vi "addBroadcastFreezeSensorValuesFrame.vi"(8 "error in (no error)":errorcluster, 9 "TriggerIRQ":bool, 10 "WaitForTrigger":bool, 11 "Subnet in":refnum<class "Subnet.lvclass">) -> (0 "error out":errorcluster, 3 "Subnet out":refnum<class "Subnet.lvclass">)   [LabVIEW 2016, in "Subnet.lvclass"]
uses:
  Subnet.lvclass
  Subnet.lvclass/Subnet.ctl
  Common_RT_Modbus/IModbus/IModbus.lvclass
  Common_RT_HPILC/HPILC/HPILC.lvclass
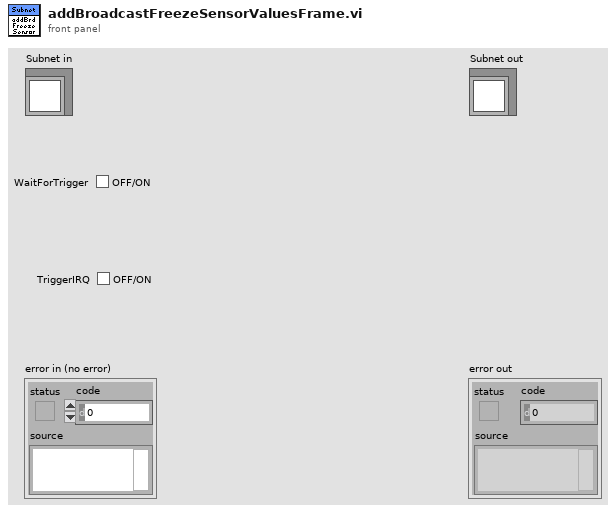
[diagram p1: front panel]
types:
  T1 = typedef "RTModbus.lvlib/TxFrame.ctl" = cluster{"Data":u8[], "WaitForTrigger":bool, "WaitForRx":u16, "TriggerIRQ":bool, "DelayMicroseconds":u16, "DelayMilliseconds":u16, "Timestamp":bool}
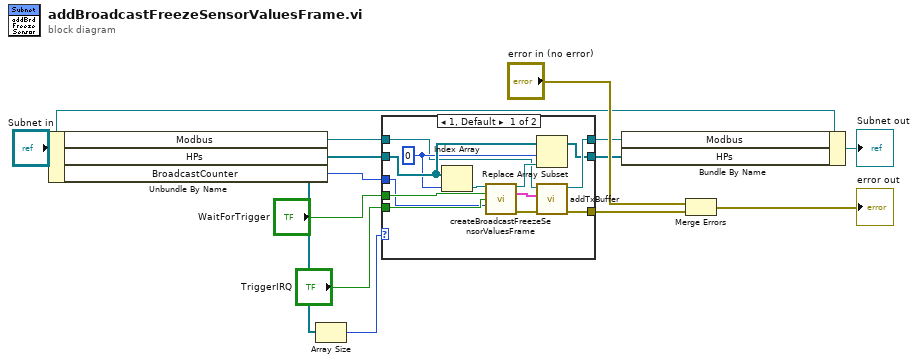
[diagram p0: block diagram]
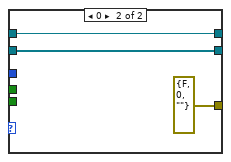
[diagram p2: hidden frame]
diagram:
  n1 = Unbundle By Name("Subnet in") -> ("Modbus"=w12:refnum<class "IModbus.lvclass">, "HPs"=w11:refnum<class "HPILC.lvclass">[], "BroadcastCounter"=w1:u8)
  n2 = Array Size(array=w11) -> (size(s)=w13:i32)
  n3 = case shown="1, Default" w13 {
    tunnel: w12 -> [w22 w28]
    tunnel: w11 -> [w25 w29]
    tunnel: [w19 errorcluster {"status"=FALSE, "code"=0, "source"=""} ("error out")] -> w10
    tunnel: [w18 w28] -> w5
    tunnel: [w17 w29] -> w4
    tunnel: "WaitForTrigger" -> [w16 _]
    tunnel: "TriggerIRQ" -> [w15 _]
    tunnel: w1 -> [w14 _]
    frame 1, Default {
      w24 = 0 ("index")
      n4 = Index Array(array=w25, index=w24) -> (element=w26:refnum<class "HPILC.lvclass">)
      n5 = call "createBroadcastFreezeSensorValuesFrame.vi"("HPILC in"=w26, "WaitForTrigger"=w16, "TriggerIRQ"=w15, "BroadcastCounter"=w14) -> ("HPILC out"=w23:refnum<class "HPILC.lvclass">, "TxFrame"=w21:T1, "error out"=w20:errorcluster)  [unwired: 9 in]
      n6 = Replace Array Subset(array=w25, new element=w23, index=w24) -> (w17:refnum<class "HPILC.lvclass">[])
      n7 = call-dynamic "addTxBuffer.vi"("error in (no error)"=w20, "TxFrame"=w21, "IModbus in"=w22) -> ("error out"=w19:errorcluster, "IModbus out"=w18:refnum<class "IModbus.lvclass">)  [unwired: 7 in]
    }
    frame 0 {
    }
  }
  n8 = Bundle By Name(cluster="Subnet in", "Modbus"=w5, "HPs"=w4) -> (→"Subnet out":refnum<class "Subnet.lvclass">)
  n9 = Merge Errors("error in (no error)", w10) -> (→"error out":errorcluster)
